vi "Result_Test.vi"(8 "error in (no error)":errorcluster caption="entrée d'erreur (pas d'erreur)", 11 "Flash_Jlink en entrée":refnum<class "Nodon_Power.lvclass">) -> (0 "error out":errorcluster caption="sortie d'erreur", 3 "Flash_Jlink en sortie":refnum<class "Nodon_Power.lvclass">)   [LabVIEW 2020, in "Library Test.lvlib" / "Nodon_Power.lvclass"]
uses:
  Nodon_Power.lvclass
  C:/Users/ngarcin/OneDrive - Altyor/Standard TB/Suite TB45/Class/Test/Test (Default)/Test (Default).lvclass
  Commun VI/TypeDef/Variable Printable.ctl
  Test_Without_Instr/Test_Without_Inst.lvclass
  Commun VI/Library Commun.lvlib
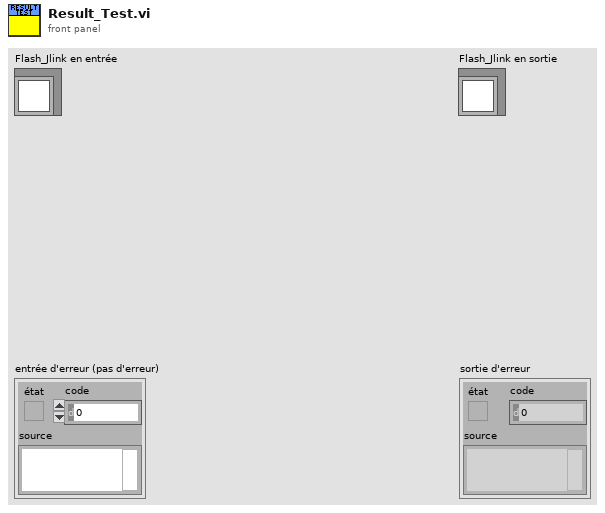
[diagram p1: front panel]
types:
  T1 = typedef "Variable Printable.ctl" = string
  T2 = enum16{"Get Variable", "Get All Variables", "Set Variable", "Delete Variable", "Delete All Variable"}
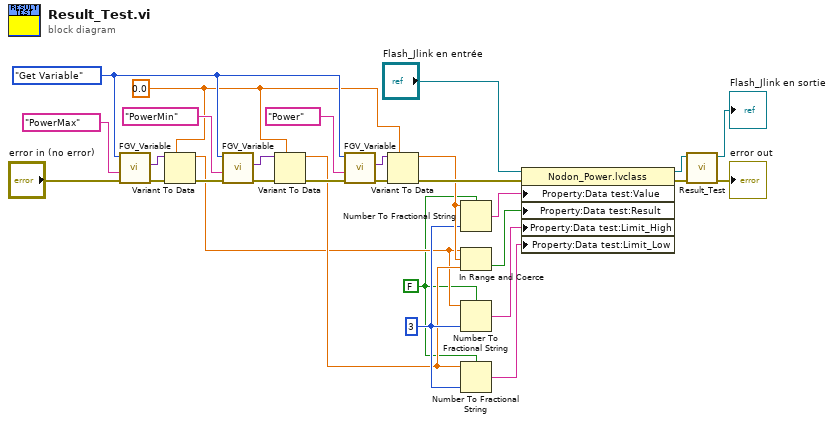
[diagram p0: block diagram]
diagram:
  w1 = FALSE ("utiliser le séparateur décimal du système (V)")
  w5 = i16 3 ("précision (6)")
  w13 = 0.0
  w22 = T2."Get Variable" ("Function")
  n1 = call "FGV_Variable.vi"("error in (no error)"="error in (no error)", "Variable"=T1 "PowerMax", "Function"=w22) -> ("error out"=w24:errorcluster, "Data Out"=w11:variant)  [unwired: 6 in, 1 out]
  n2 = Variant To Data(error in=w24, type=w13, Variant=w11) -> (data=w2:dbl, error out=w19:errorcluster)
  n3 = call "FGV_Variable.vi"("error in (no error)"=w19, "Variable"=T1 "PowerMin", "Function"=w22) -> ("error out"=w23:errorcluster, "Data Out"=w12:variant)  [unwired: 6 in, 1 out]
  n4 = Variant To Data(error in=w23, type=w13, Variant=w12) -> (data=w3:dbl, error out=w18:errorcluster)
  n5 = call "FGV_Variable.vi"("error in (no error)"=w18, "Variable"=T1 "Power", "Function"=w22) -> ("error out"=w17:errorcluster, "Data Out"=w15:variant)  [unwired: 6 in, 1 out]
  n6 = Variant To Data(error in=w17, type=w13, Variant=w15) -> (data=w10:dbl, error out=w16:errorcluster)
  n7 = Number To Fractional String(use system decimal point (T)=w1, number=w10, precision (6)=w5) -> (F-format string=w9:string)  [unwired: 1 in]
  n8 = In Range and Coerce(upper limit=w2, x=w10, lower limit=w3) -> (In Range?=w14:bool)  [unwired: 1 out]
  n9 = Number To Fractional String(use system decimal point (T)=w1, number=w2, precision (6)=w5) -> (F-format string=w6:string)  [unwired: 1 in]
  n10 = Number To Fractional String(use system decimal point (T)=w1, number=w3, precision (6)=w5) -> (F-format string=w4:string)  [unwired: 1 in]
  n11 = property class="Nodon_Power.lvclass"(reference="Flash_Jlink en entrée", error in=w16, "Property:Data test:Value"=w9, "Property:Data test:Result"=w14, "Property:Data test:Limit_High"=w6, "Property:Data test:Limit_Low"=w4) -> (reference out=w26:refnum<class "Nodon_Power.lvclass">, error out=w27:errorcluster)
  n12 = call-parent "Result_Test.vi"("error in (no error)"=w27, "Test_Without_Inst en entrée"=w26) -> ("error out"=→"error out":errorcluster, "Test_Without_Inst en sortie"=→"Flash_Jlink en sortie":refnum<class "Nodon_Power.lvclass">)  [unwired: 8 in]
